vi "queryGap.vi"(0 "连接ID":refnum<k5>) -> (1 "连接ID输出":refnum<k5>, 2 "gap":dbl, 3 "gap speed":dbl, 4 "z home speed":dbl)   [LabVIEW 2017]
uses:
  <vilib>/LVH/i3 JSON/JSON Parsing/Get Object Parameter Files/Get Object Parameter - Numeric.vi
  <vilib>/LVH/i3 JSON/i3-json.lvlib
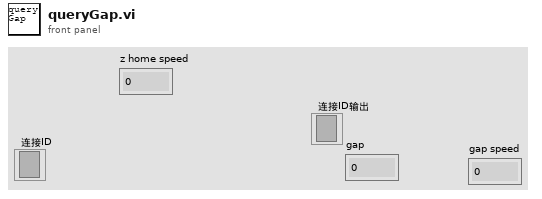
[diagram p1: front panel]
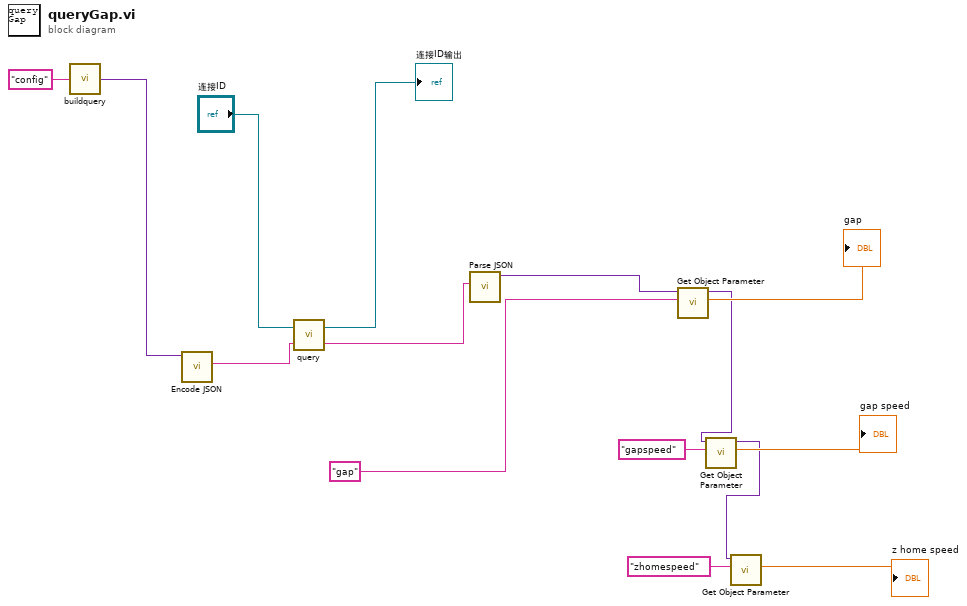
[diagram p0: block diagram]
diagram:
  n1 = call "buildquery.vi"("String"="config") -> ("JSON Tree out (JSON Object)"=w10:variant)
  n2 = call <vilib>:"Encode JSON.vi"("JSON Tree"=w10) -> ("String"=w14:string)  [unwired: 5 in, 1 out]
  n3 = call "query.vi"("数据输入"=w14, "连接ID"="连接ID") -> ("数据输出"=w12:string, "连接ID输出"=→"连接ID输出":refnum<k5>)
  n4 = call <vilib>:"Parse JSON.vi"("JSON String"=w12) -> ("JSON Tree"=w11:variant)  [unwired: 7 in, 3 out]
  n5 = call-poly <vilib>:"Get Object Parameter.vi"("Parameter Name"="gap", "JSON Tree In (JSON Object)"=w11) -> ("Double Value"=→"gap":dbl, "JSON Tree Out Passthrough"=w6:variant)  [unwired: 6 in, 2 out]
  n6 = call-poly <vilib>:"Get Object Parameter.vi"("Parameter Name"="gapspeed", "JSON Tree In (JSON Object)"=w6) -> ("Double Value"=→"gap speed":dbl, "JSON Tree Out Passthrough"=w2:variant)  [unwired: 6 in, 2 out]
  n7 = call-poly <vilib>:"Get Object Parameter.vi"("Parameter Name"="zhomespeed", "JSON Tree In (JSON Object)"=w2) -> ("Double Value"=→"z home speed":dbl)  [unwired: 6 in, 3 out]
